vi "resistanceDisplay.vi"(0 "refnum in":refnum<file>, 1 "resistanceMin":u32, 2 "resistanceMid":u32, 3 "resistanceMax":u32, 5 "VISA resource name":refnum<visa-resource-name>, 7 "write buffer buffer":string="G\u0002", 9 "E-Stop/Incline":bool, 11 "error in":errorcluster) -> (4 "RESISTANCE/CURRENT":cluster{"number[0]":u32, dbl}(graph), 6 "resultIncline":bool, 8 "resistance#":u32, 10 "current#":string, 15 "error out":errorcluster)   [LabVIEW 2018]
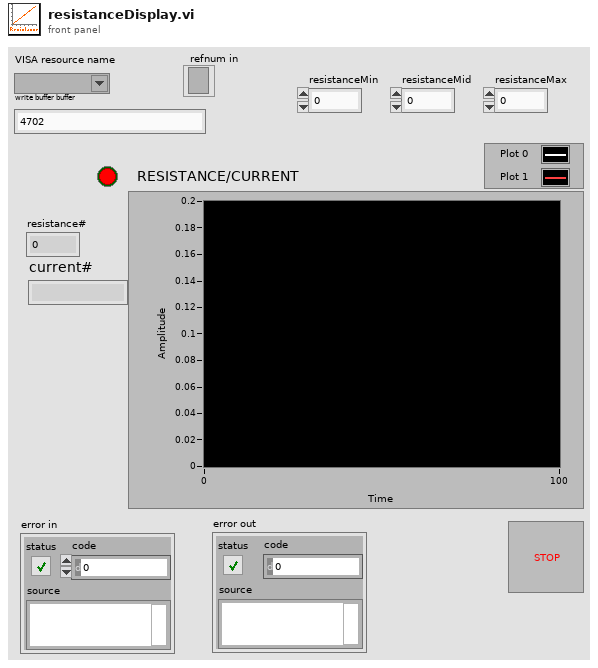
[diagram p1: front panel]
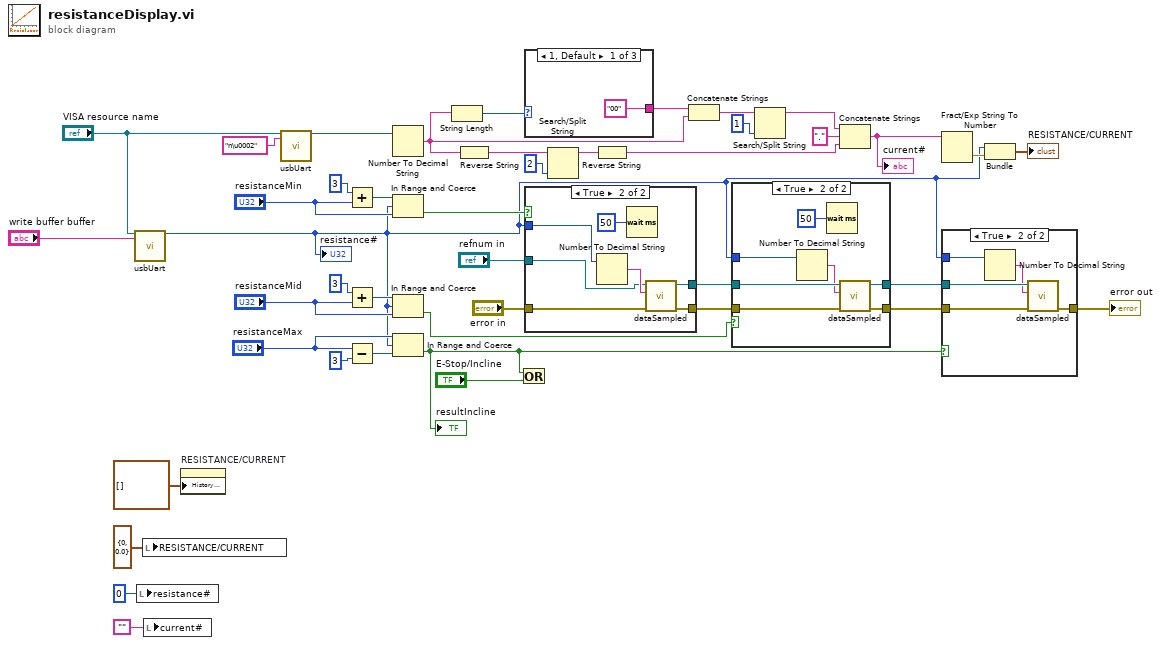
[diagram p0: block diagram]
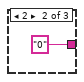
[diagram p2: hidden frame]
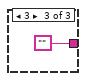
[diagram p3: hidden frame]
diagram:
  n1 = call "usbUart.vi"("VISA resource name"="VISA resource name", "write buffer"="write buffer buffer") -> ("number[0]"=w1:u32)  [unwired: 2 in, 15 out]
  "resistance#" <- w1
  n2 = local write "resistance#"(u32 0 ("resistance#")) -> ()
  n3 = local write "RESISTANCE/CURRENT"(cluster{"number[0]":u32, dbl} {"number[0]"=0, 0.0} ("RESISTANCE/CURRENT")) -> ()
  n4 = local write "current#"("") -> ()
  n5 = property on="RESISTANCE/CURRENT" class="WFChart (strict)"("History Data"=cluster{"number[0]":u32, dbl}[] []) -> ()  [unwired: 2 in, 2 out]
  n6 = call "usbUart.vi"("VISA resource name"="VISA resource name", "write buffer"="n\u0002") -> ("number[0]"=w25:u32)  [unwired: 2 in, 15 out]
  n7 = Add(x=u32 3, y="resistanceMin") -> (x+y=w8:u32)
  n8 = Add(x=u32 3, y="resistanceMid") -> (x+y=w6:u32)
  n9 = Subtract(x="resistanceMax", y=u32 3) -> (x-y=w2:u32)
  n10 = Number To Decimal String(number=w25) -> (decimal integer string=w23:string)  [unwired: 1 in]
  n11 = In Range and Coerce(upper limit=w8, x=w1, lower limit="resistanceMin") -> (In Range?=w34:bool)  [unwired: 1 out]
  n12 = In Range and Coerce(upper limit=w6, x=w1, lower limit="resistanceMid") -> (In Range?=w29:bool)  [unwired: 1 out]
  n13 = In Range and Coerce(upper limit="resistanceMax", x=w1, lower limit=w2) -> (In Range?=w27:bool)  [unwired: 1 out]
  "resultIncline" <- w27
  n14 = String Length(string=w23) -> (length=w21:i32)
  n15 = Reverse String(1:w23) -> (0:w17:string)
  n16 = Or(x=w27, y="E-Stop/Incline") -> ()  [unwired: 1 out]
  n17 = case shown="1, Default" w21 {
    tunnel: ["00" "0" ""] -> w22
    frame 1, Default {
    }
    frame 2 {
    }
    frame 3 {
    }
  }
  n18 = case shown="True" w34 {
    tunnel: "error in" -> [w48 w55]
    tunnel: w1 -> [_ w53]
    tunnel: [w47 w52] -> w33
    tunnel: [w48 w51] -> w32
    tunnel: "refnum in" -> [w47 w49]
    frame False {
    }
    frame True {
      n19 = Number To Decimal String(number=w53) -> (decimal integer string=w54:string)  [unwired: 1 in]
      n20 = Wait (ms)(milliseconds to wait=u32 50) -> ()  [unwired: 1 out]
      n21 = call "dataSampled.vi"("Error In"=w55, "Data"=w54, "refnum in"=w49) -> ("error out"=w51:errorcluster, "refnum out"=w52:refnum<file>)  [unwired: 7 in]
    }
  }
  n22 = Search/Split String(string=w17, offset (0)=2) -> (substring before match=w18:string)  [unwired: 1 in, 2 out]
  n23 = Reverse String(1:w18) -> (0:w20:string)
  n24 = Concatenate Strings(w22, w23) -> (w24:string)
  n25 = case shown="True" w29 {
    tunnel: w33 -> [w57 w64]
    tunnel: w32 -> [w56 w63]
    tunnel: w1 -> [_ w61]
    tunnel: [w57 w60] -> w31
    tunnel: [w56 w59] -> w30
    frame False {
    }
    frame True {
      n26 = Number To Decimal String(number=w61) -> (decimal integer string=w62:string)  [unwired: 1 in]
      n27 = Wait (ms)(milliseconds to wait=u32 50) -> ()  [unwired: 1 out]
      n28 = call "dataSampled.vi"("Error In"=w63, "Data"=w62, "refnum in"=w64) -> ("error out"=w59:errorcluster, "refnum out"=w60:refnum<file>)  [unwired: 7 in]
    }
  }
  n29 = Search/Split String(string=w24, offset (0)=1) -> (substring before match=w19:string)  [unwired: 1 in, 2 out]
  n30 = Concatenate Strings(w19, "." ("string"), w20) -> (w12:string)
  "current#" <- w12
  n31 = Fract/Exp String To Number(string=w12) -> (number=w11:dbl)  [unwired: 3 in, 1 out]
  n32 = case shown="True" w27 {
    tunnel: w31 -> [_ w70]
    tunnel: w30 -> [w65 w69]
    tunnel: w1 -> [_ w67]
    tunnel: [w65 w66] -> w41
    frame False {
    }
    frame True {
      n33 = Number To Decimal String(number=w67) -> (decimal integer string=w68:string)  [unwired: 1 in]
      n34 = call "dataSampled.vi"("Error In"=w69, "Data"=w68, "refnum in"=w70) -> ("error out"=w66:errorcluster)  [unwired: 7 in, 1 out]
    }
  }
  "error out" <- w41
  n35 = Bundle("number[0]"=w1, w11) -> (→"RESISTANCE/CURRENT":cluster{"number[0]":u32, dbl})  [unwired: 1 in]
